vi "SubVI_RampTesting_Teleop.vi"(8 "error in (no error)":errorcluster, 10 "threshold":dbl=0.1 format="%#_14g", 11 "Y Input":dbl) -> (0 "error out":errorcluster, 3 "Y Output":dbl)   [LabVIEW 2017]
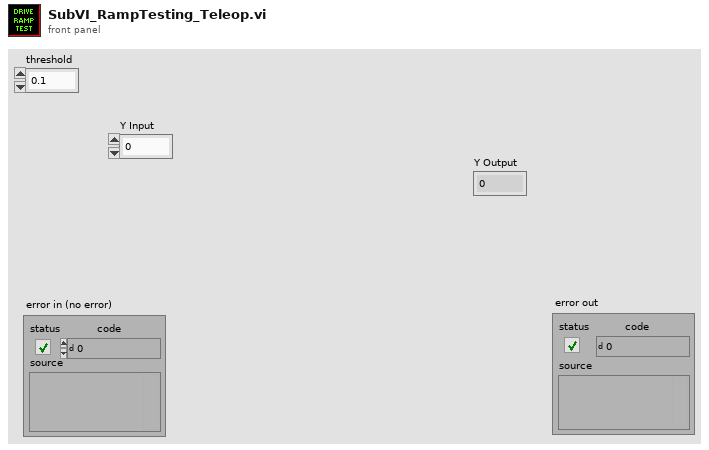
[diagram p1: front panel]
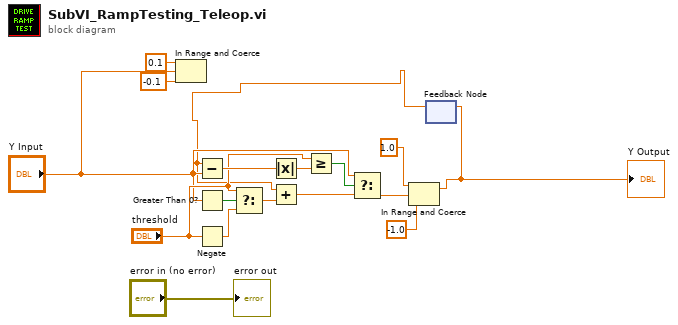
[diagram p0: block diagram]
diagram:
  n1 = In Range and Coerce(upper limit=0.1, x="Y Input", lower limit=-0.1) -> ()  [unwired: 2 out]
  n2 = Greater Than 0?(x="Y Input") -> (x > 0?=w12:bool)
  n3 = Negate(x="threshold") -> (-x=w10:dbl)
  n4 = Select(t="threshold", s=w12, f=w10) -> (s? t:f=w9:dbl)
  n5 = feedback #1() -> (w1:dbl)  [unwired: 1 in]
  n6 = Subtract(x=w1, y="Y Input") -> (x-y=w15:dbl)
  n7 = Absolute Value(x=w15) -> (abs(x)=w14:dbl)
  n8 = Add(x=w1, y=w9) -> (x+y=w8:dbl)
  n9 = Greater Or Equal?(x="threshold", y=w14) -> (x >= y?=w13:bool)
  n10 = Select(t="Y Input", s=w13, f=w8) -> (s? t:f=w5:dbl)
  n11 = In Range and Coerce(upper limit=1.0, x=w5, lower limit=-1.0) -> (coerced(x)=w16:dbl)  [unwired: 1 out]
  "Y Output" <- w16
  n12 = feedback-in #1(w16) -> ()
  "error out" <- "error in (no error)"
